vi "Wait for Button.vi"(11 "IO":T1) -> (3 "bt_Node out":refnum<class "bt_Node.lvclass">)   [LabVIEW 2021, in "Test Sequencer Support.lvlib"]
uses:
  Test Sequencer Support.lvlib
  Support/Nodes/abs_Node/bt_Node.lvclass
  IO Type.ctl
  <vilib>/TSA/Event Log/Event_TextLog/Event_TextLog.lvclass
  Blackboard/Blackboard.lvclass
  <vilib>/TSA/Abstract Data Classes/Abs_Types/Boolean/Abs_Boolean.lvclass
  C:/Program Files (x86)/National Instruments/LabVIEW 2021/vi.lib/TSA/Abstract Data Classes/Abs_Types/Value/Abs_Value.lvclass
  C:/Program Files (x86)/National Instruments/LabVIEW 2021/vi.lib/TSA/Abstract Data Classes/Abs_Types/Type/Abs_Type.lvclass
  <vilib>/TSA/Abstract Data Classes/Abs_Types/Waveform/Abs_Waveform.lvclass
  <vilib>/TSA/Abstract Data Classes/Abs_Types/Double Float/Abs_Double Float.lvclass
  Support/Nodes/Decorators/Repeater/Support/Finish On - Type.ctl
  Support/Nodes/Leaves/abs_Type Leaf/abs_Type Leaf.lvclass/abs_Type Leaf.ctl
  Support/Nodes/Leaves/abs_Type Leaf/Properties/Write Value Class.vi
  Support/Nodes/Leaves/Test Boolean/Test Abs_Boolean.lvclass
  C:/Users/timst/Documents/Repositories/LV_Behaviour_Tree/Source/Support/Nodes/abs_Node/bt_Node.lvclass
  C:/Users/timst/Documents/Repositories/LV_Behaviour_Tree/Source/Support/Nodes/Leaves/abs_Type Leaf/abs_Type Leaf.lvclass
  <vilib>/TSA/Abstract Data Classes/Constants/Support/Bool/Bool.vi
  BT.lvlib
  Support/Nodes/Decorators/Repeater/bt_Repeater.lvclass
  <vilib>/TSA/Abstract Data Classes/Constants/Support/Bool/Const_Bool.lvclass
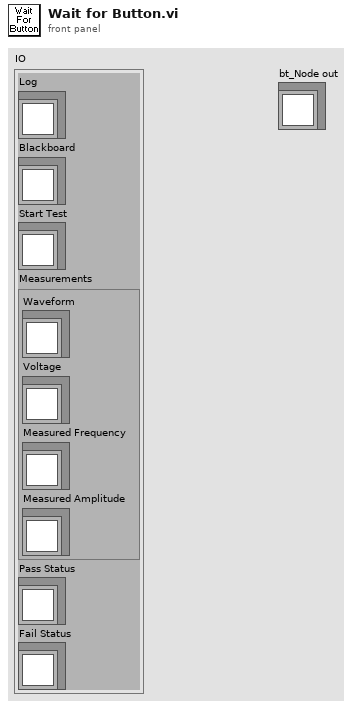
[diagram p1: front panel]
types:
  T1 = typedef "Test Sequencer Support.lvlib/IO Type.ctl" = cluster{"Log":refnum<class "Event_TextLog.lvclass">, "Blackboard":refnum<class "Blackboard.lvclass">, "Start Test":refnum<class "Abs_Boolean.lvclass">, "Measurements":cluster{"Waveform":refnum<class "Abs_Waveform.lvclass">, "Voltage":refnum<class "Abs_Double Float.lvclass">, "Measured Frequency":refnum<class "Abs_Double Float.lvclass">, "Measured Amplitude":refnum<class "Abs_Double Float.lvclass">}, "Pass Status":refnum<class "Abs_Boolean.lvclass">, "Fail Status":refnum<class "Abs_Boolean.lvclass">}
  T2 = typedef "BT.lvlib/bt_Repeater.lvclass/Finish On - Type.ctl" = enum16{"Success", "Failure", "Never"}
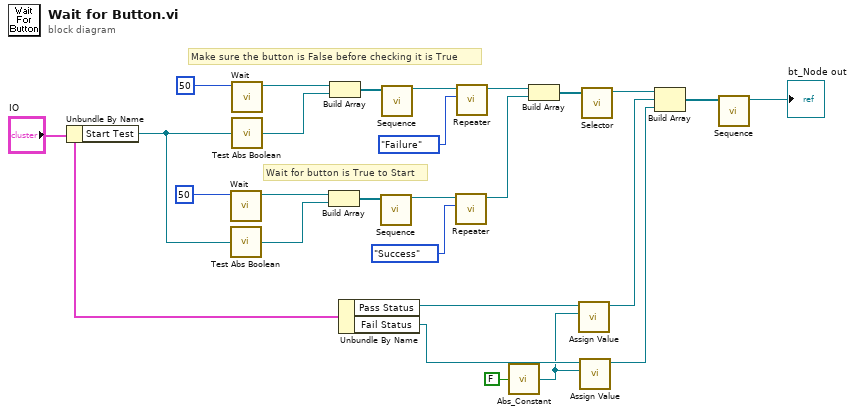
[diagram p0: block diagram]
diagram:
  # "Wait for button is True to Start"
  # "Make sure the button is False before checking it is True"
  n1 = Unbundle By Name("IO") -> ("Start Test"=w9:refnum<class "Abs_Boolean.lvclass">)
  n2 = call "Wait.vi"("Time (ms)"=u32 50) -> ("Node Out"=w23:refnum<class "bt_Node.lvclass">)  [unwired: 10 in]
  n3 = call "Test Abs Boolean.vi"("Abs_Boolean.lvclass"=w9) -> ("abs_Node"=w24:refnum<class "bt_Node.lvclass">)  [unwired: 4 in]
  n4 = call "Wait.vi"("Time (ms)"=u32 50) -> ("Node Out"=w18:refnum<class "bt_Node.lvclass">)  [unwired: 10 in]
  n5 = call "Test Abs Boolean.vi"("Abs_Boolean.lvclass"=w9) -> ("abs_Node"=w17:refnum<class "bt_Node.lvclass">)  [unwired: 4 in]
  n6 = Build Array(w23, w24) -> (w25:refnum<class "bt_Node.lvclass">[])
  n7 = Build Array(w18, w17) -> (w16:refnum<class "bt_Node.lvclass">[])
  n8 = Unbundle By Name("IO") -> ("Pass Status"=w7:refnum<class "Abs_Boolean.lvclass">, "Fail Status"=w5:refnum<class "Abs_Boolean.lvclass">)
  n9 = call "Sequence.vi"("Nodes"=w25) -> ("Node"=w21:refnum<class "bt_Node.lvclass">)  [unwired: 10 in]
  n10 = call "Sequence.vi"("Nodes"=w16) -> ("Node"=w20:refnum<class "bt_Node.lvclass">)  [unwired: 10 in]
  n11 = call "Repeater.vi"("Finish On"=Finish_On_-_Type."Success", "Node In"=w21) -> ("Node Out"=w13:refnum<class "bt_Node.lvclass">)  [unwired: 9 in]
  n12 = call "Repeater.vi"("Finish On"=Finish_On_-_Type."Failure", "Node In"=w20) -> ("Node Out"=w14:refnum<class "bt_Node.lvclass">)  [unwired: 9 in]
  n13 = call-poly <vilib>:"Abs_Constant.vi"("Boolean"=FALSE) -> ("Abs_Boolean.lvclass"=w3:refnum<class "Abs_Boolean.lvclass">)  [unwired: 4 in]
  n14 = Build Array(w14, w13) -> (w12:refnum<class "bt_Node.lvclass">[])
  n15 = call "Assign Value.vi"("Assigned Value"=w3, "Value"=w7) -> ("Node Out"=w10:refnum<class "bt_Node.lvclass">)  [unwired: 9 in]
  n16 = call "Assign Value.vi"("Assigned Value"=w3, "Value"=w5) -> ("Node Out"=w6:refnum<class "bt_Node.lvclass">)  [unwired: 9 in]
  n17 = call "Selector.vi"("Nodes"=w12) -> ("Node"=w1:refnum<class "bt_Node.lvclass">)  [unwired: 10 in]
  n18 = Build Array(w1, w10, w6) -> (w11:refnum<class "bt_Node.lvclass">[])
  n19 = call "Sequence.vi"("Nodes"=w11) -> ("Node"=→"bt_Node out":refnum<class "bt_Node.lvclass">)  [unwired: 10 in]
